vi "SOAE-Restore Defaults.vi"() -> (4 "Params":T3, 8 "Options":T1, 15 "error out":errorcluster)   [LabVIEW 2020]
uses:
  Utility VIs/Type Defs/Left-Right ring.ctl
  Typedefs/SOAE-Options.ctl
panel:
  in  "Default options":T1={"FreqScale"={"Min"=4000.0, "Max"=48000.0}, "save raw"=FALSE}
  in  "Default params":T3={"Ear"=enum."Right", "Fs (Hz)"=100000.0, "Nfft"=546448, "Number of averages"=40.0, "Binwidth (Hz)"=93.0, "Gain (dB)"=40.0}
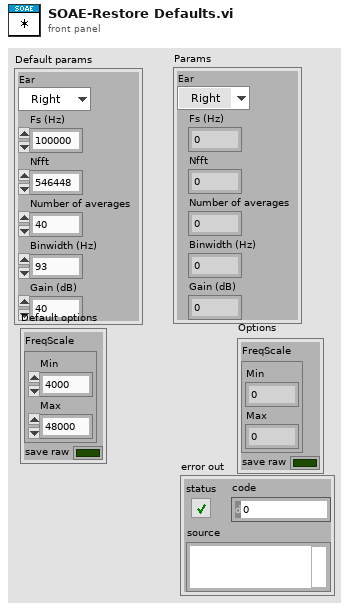
[diagram p1: front panel]
types:
  T1 = typedef "SOAE-Options.ctl" = cluster{"FreqScale":cluster{"Min":dbl, "Max":dbl}, "save raw":bool}
  T2 = typedef "Left-Right ring.ctl" = enum16{"Right", "Left"}
  T3 = cluster{"Ear":T2, "Fs (Hz)":dbl, "Nfft":i32, "Number of averages":dbl, "Binwidth (Hz)":dbl, "Gain (dB)":dbl}
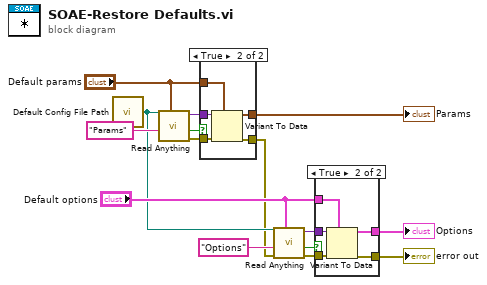
[diagram p0: block diagram]
diagram:
  n1 = call "Default Config File Path.vi"() -> ("Default config file name"=w3:path)
  n2 = call "Read Anything.vi"("Type of Anything"="Default params", "Section Name (Name of \"Type of Anything\")"="Params" ("Section Name (Name of \"Type of Anything\")"), "Path (dialog)"=w3) -> ("Error Out"=w11:errorcluster, "Found?"=w13:bool, "Anything"=w12:variant)  [unwired: 6 in]
  n3 = case shown="True" w13 {
    tunnel: w11 -> [w16 w22]
    tunnel: w12 -> [_ w21]
    tunnel: [w17 w20] -> w15
    tunnel: [w16 w19] -> w2
    tunnel: "Default params" -> [w17 w18]
    frame False {
    }
    frame True {
      n4 = Variant To Data(error in=w22, type=w18, Variant=w21) -> (data=w20:T3, error out=w19:errorcluster)
    }
  }
  "Params" <- w15
  n5 = call "Read Anything.vi"("Type of Anything"="Default options", "Error In"=w2, "Section Name (Name of \"Type of Anything\")"="Options" ("Section Name (Name of \"Type of Anything\")"), "Path (dialog)"=w3) -> ("Error Out"=w7:errorcluster, "Found?"=w9:bool, "Anything"=w8:variant)  [unwired: 5 in]
  n6 = case shown="True" w9 {
    tunnel: w7 -> [w23 w29]
    tunnel: w8 -> [_ w28]
    tunnel: [w24 w27] -> w4
    tunnel: [w23 w26] -> w1
    tunnel: "Default options" -> [w24 w25]
    frame False {
    }
    frame True {
      n7 = Variant To Data(error in=w29, type=w25, Variant=w28) -> (data=w27:T1, error out=w26:errorcluster)
    }
  }
  "error out" <- w1
  "Options" <- w4
